vi "example.vi"() -> ()   [LabVIEW 2019]
uses:
  <vilib>/httpClient/POSTBuffer.vi
  <vilib>/httpClient/LabVIEWHTTPClient.lvlib
panel:
  in  "Target Path":string="c:\\"
  in  "Source URL":string="http://192.168.12.1/cgi-bin/pleaseGiveMeAFile?location=mmcblk1p1&fileName="
  in  "Copy from SD card to computer":bool
  out "Filename":string
  out "HTTP Response - save video":string
  out "HTTP response - apply resolution":string
  in  "Save Video to SD card in camera":bool
  in  "Apply Resolution":bool
  in  "Height":dbl
  in  "Width":dbl
  in  "Stop Recording":bool
  in  "Start Recording":bool
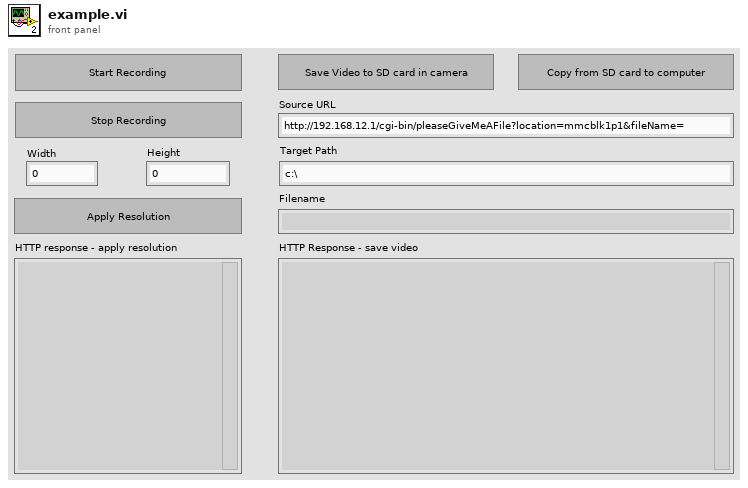
[diagram p1: front panel]
types:
  T1 = typedef "LabVIEWHTTPClient.lvlib/ClientHandle.ctl" = refnum<k1>
  T2 = enum16{"open", "open or create", "create or replace", "create", "open (read only)"}
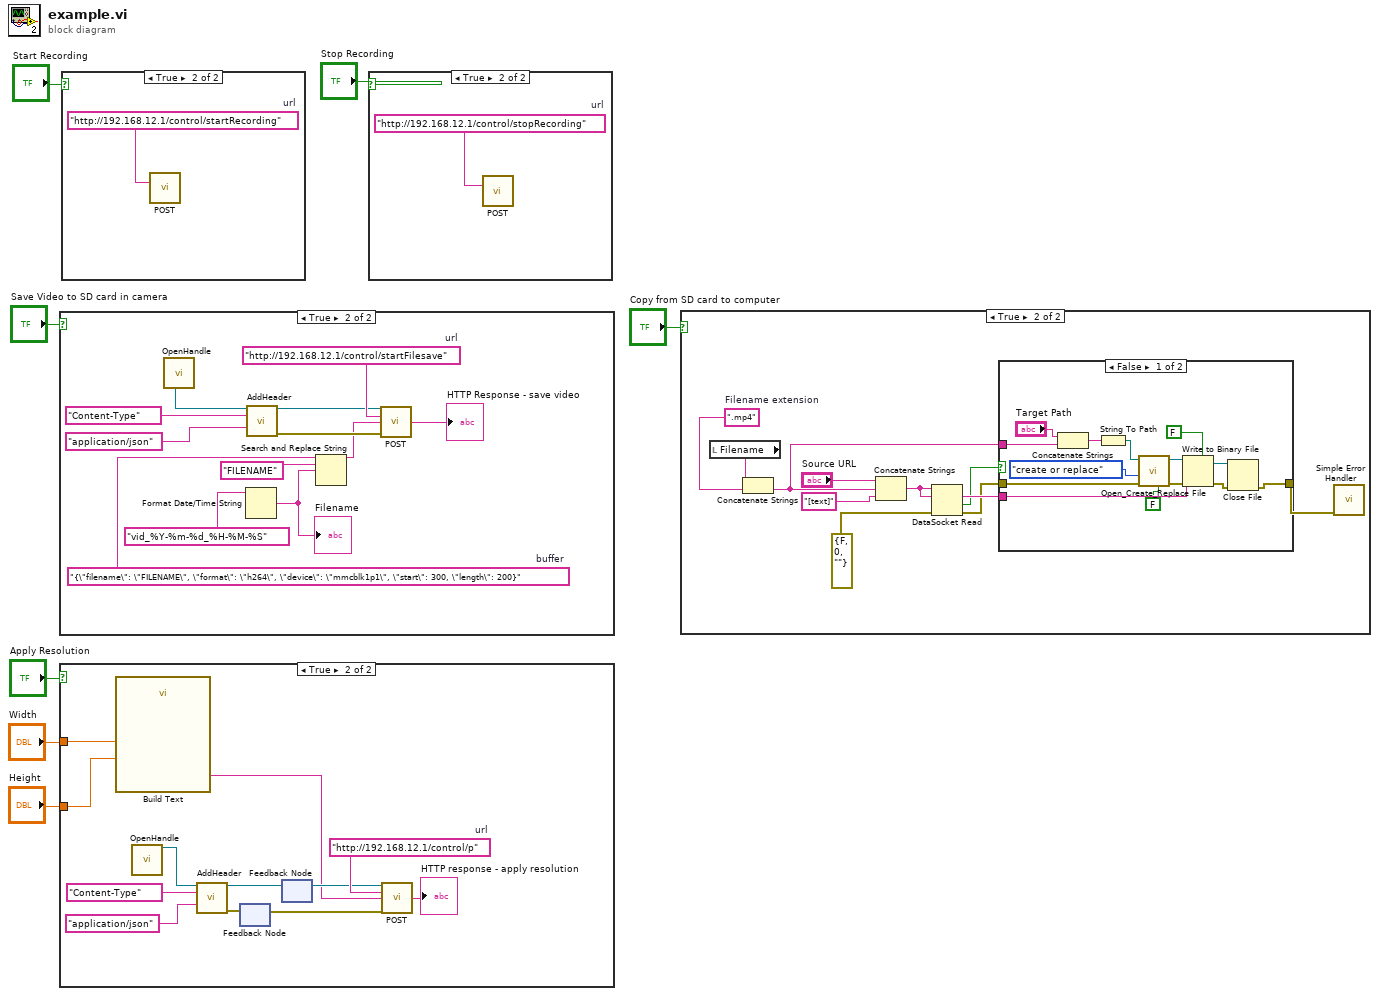
[diagram p0: block diagram]
diagram:
  n1 = case shown="True" "Save Video to SD card in camera" {
    frame False {
    }
    frame True {
      w12 = "{\"filename\": \"FILENAME\", \"format\": \"h264\", \"device\": \"mmcblk1p1\", \"start\": 300, \"length\": 200}"  # buffer
      w19 = "http://192.168.12.1/control/startFilesave"  # url
      n2 = call <vilib>:"OpenHandle.vi"() -> ("client handle out"=w17:T1)  [unwired: 14 in, 1 out]
      n3 = Format Date/Time String(time format string (%c)="vid_%Y-%m-%d_%H-%M-%S") -> (date/time string=w8:string)  [unwired: 2 in]
      "Filename" <- w8
      n4 = call <vilib>:"AddHeader.vi"("client handle"=w17, "header"="Content-Type", "value"="application/json") -> ("client handle out"=w14:T1, "error out"=w13:errorcluster)  [unwired: 11 in]
      n5 = Search and Replace String(input string=w12, search string="FILENAME", replace string=w8) -> (result string=w10:string)  [unwired: 5 in, 3 out]
      n6 = call-poly <vilib>:"POST.vi"("client handle"=w14, "url"=w19, "buffer"=w10, "error in (no error)"=w13) -> ("body"=→"HTTP Response - save video":string)  [unwired: 8 in, 3 out]
    }
  }
  n7 = case shown="True" "Apply Resolution" {
    tunnel: "Height" -> [_ w21]
    tunnel: "Width" -> [_ w20]
    frame False {
    }
    frame True {
      w31 = "http://192.168.12.1/control/p"  # url
      n8 = call "Build Text"("HRES"=w20, "VRES"=w21) -> ("Result"=w22:string)  [unwired: 12 in, 1 out]
      n9 = call <vilib>:"OpenHandle.vi"() -> ("client handle out"=w28:T1)  [unwired: 14 in, 1 out]
      n10 = call <vilib>:"AddHeader.vi"("client handle"=w28, "header"="Content-Type", "value"="application/json") -> ("client handle out"=w27:T1, "error out"=w30:errorcluster)  [unwired: 11 in]
      n11 = feedback-in #1(w30) -> ()
      n12 = feedback #1() -> (w29:errorcluster)  [unwired: 1 in]
      n13 = feedback-in #2(w27) -> ()
      n14 = feedback #2() -> (w26:T1)  [unwired: 1 in]
      n15 = call-poly <vilib>:"POST.vi"("client handle"=w26, "url"=w31, "buffer"=w22, "error in (no error)"=w29) -> ("body"=→"HTTP response - apply resolution":string)  [unwired: 8 in, 3 out]
    }
  }
  n16 = case shown="True" "Start Recording" {
    frame False {
    }
    frame True {
      w32 = "http://192.168.12.1/control/startRecording"  # url
      n17 = call-poly <vilib>:"POST.vi"("url"=w32) -> ()  [unwired: 11 in, 4 out]
    }
  }
  n18 = case shown="True" "Stop Recording" {
    frame False {
    }
    frame True {
      w33 = "http://192.168.12.1/control/stopRecording"  # url
      n19 = call-poly <vilib>:"POST.vi"("url"=w33) -> ()  [unwired: 11 in, 4 out]
    }
  }
  n20 = case shown="True" "Copy from SD card to computer" {
    frame False {
    }
    frame True {
      w35 = ".mp4"  # Filename extension
      n21 = local read "Filename"() -> (w36:string)
      n22 = Concatenate Strings(w36, w35) -> (w34:string)
      n23 = Concatenate Strings("Source URL", w34, "[text]" ("string")) -> (w42:string)
      n24 = DataSocket Read(8:errorcluster {"status"=FALSE, "code"=0, "source"=""} ("error out"), 10:w42, 11:w42) -> (0:w38:errorcluster, 1:w37:bool, 2:w39:string)  [unwired: 2 in, 4 out]
      n25 = case shown="False" w37 {
        tunnel: w39 -> [w58 _]
        tunnel: w34 -> [w48 _]
        tunnel: w38 -> [w47 w59]
        tunnel: [w46 w59] -> w44
        frame False {
          n26 = Concatenate Strings("Target Path", w48) -> (w49:string)
          n27 = String To Path(string=w49) -> (path=w51:path)
          n28 = call <vilib>:"Open_Create_Replace File.vi"("advisory dialog? (display:T)"=FALSE, "error in (no error)"=w47, "function (open:0)"=T2."create or replace", "file path"=w51) -> ("error out"=w53:errorcluster, "refnum"=w57:refnum<file>)  [unwired: 4 in, 2 out]
          n29 = Write to Binary File(file (use dialog)=w57, data=w58, error in=w53, 5:FALSE ("prepend array or string size? (T)")) -> (refnum out=w56:refnum<file>, error out=w55:errorcluster)  [unwired: 2 in, 1 out]
          n30 = Close File(refnum=w56, error in=w55) -> (error out=w46:errorcluster)  [unwired: 1 out]
        }
        frame True {
        }
      }
      n31 = call <vilib>:"Simple Error Handler.vi"("error in (no error)"=w44) -> ()  [unwired: 4 in, 5 out]
    }
  }
